vi "rydberg_synth_vi.vi"(8 "error in (no error)":errorcluster, 10 "Novatech Synth Settings":T1[][](array[typedef]) {"Table Mode"."Freq. Step (MHz)" format="%#_9g"; "Table Mode"."FinalFreq" format="%#_9g"; "Table Mode"."Initial Freq.(MHz)" format="%#_9g"; "Channel Settings"."Frequency (MHz)" format="%#_9g"}) -> (0 "error out":errorcluster)   [LabVIEW 2016]
uses:
  Controls/Synth_409b/Synth_controls.ctl
  Controls/Synth_409b/synth_channel.ctl
  Controls/Synth_409b/table_mode.ctl
  <vilib>/Instr/_visa.llb/VISA Configure Serial Port (Instr).vi
panel:
  out "Response":string
  out "Whole Command":string
  # "Red Sat Abs Control - Com 6\nChannel 0: 81.85\nChannel 1: 82.15"
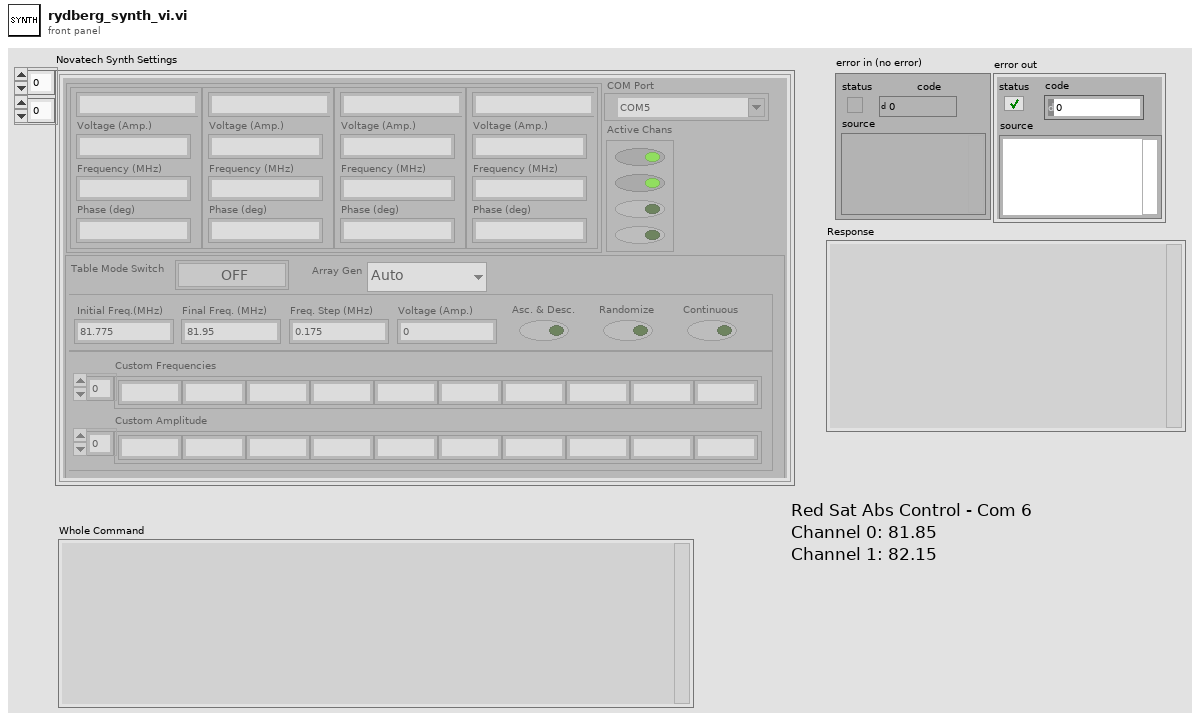
[diagram p1: front panel]
types:
  T1 = typedef "Synth_controls.ctl" = cluster{"Channel Settings":T2[], "Active Chans":bool[], "COM Port":refnum<visa-resource-name>, "Table Mode":T3}
  T2 = typedef "synth_channel.ctl" = cluster{"Voltage (Amp.) ":dbl, "Frequency (MHz)":dbl, "Phase (deg)":dbl, "Nickname":string}
  T3 = typedef "table_mode.ctl" = cluster{"Initial Freq.(MHz)":dbl, "FinalFreq":dbl, "Freq. Step (MHz)":dbl, "Voltage (Amp.)":dbl, "Asc. & Desc.":bool, "Custom Frequencies":dbl[], "Custom Amplitude":dbl[], "Table Mode Switch":bool, "Array Gen":enum16{"Auto", "Custom"}, "Randomize":bool, "Continuous":bool}
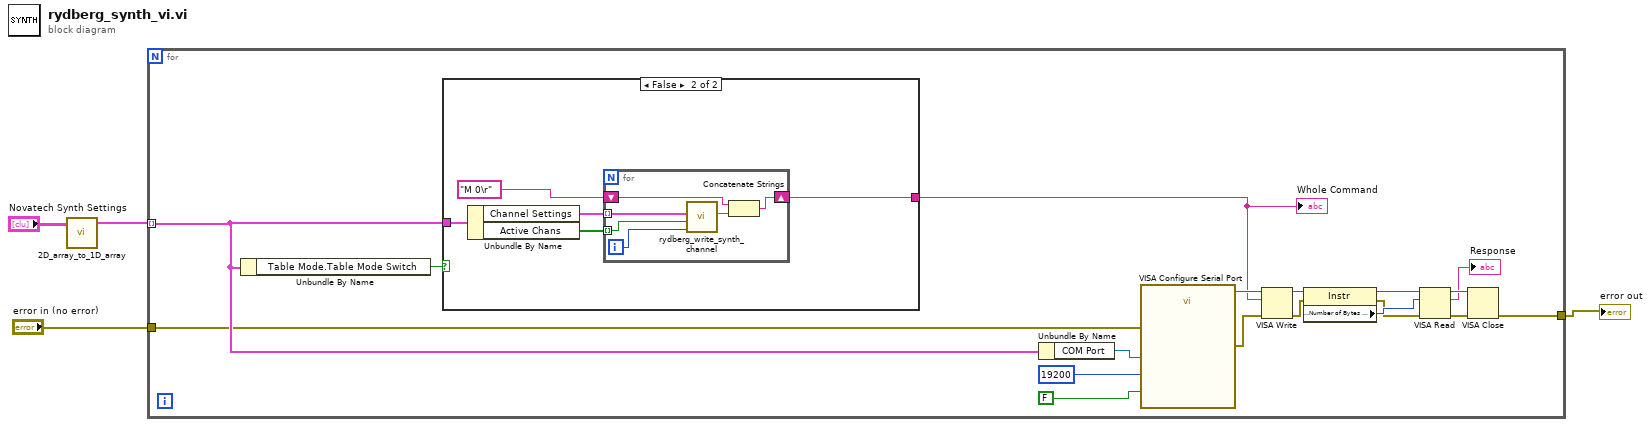
[diagram p0: block diagram]
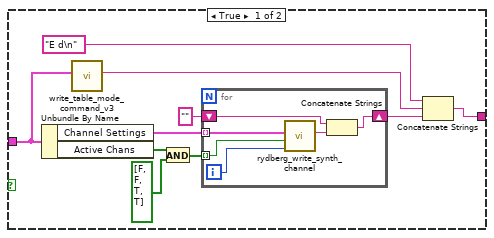
[diagram p2: hidden frame]
diagram:
  n1 = call "2D_array_to_1D_array.vi"("2D Input Arrray"="Novatech Synth Settings") -> ("1D Output array"=w1:T1[])  [unwired: 2 in, 2 out]
  n2 = for {
    tunnel: w1 -> [w7] mode=indexing
    tunnel: "error in (no error)" -> [w6]
    tunnel: [w5] -> w3
    n3 = Unbundle By Name(w7) -> ("Table Mode.Table Mode Switch"=w8:bool)
    n4 = case shown="False" w8 {
      tunnel: w7 -> [w32 w43]
      tunnel: [w29 w39] -> w10
      frame True {
        n5 = Unbundle By Name(w32) -> ("Channel Settings"=w31:T2[], "Active Chans"=w27:bool[])
        n6 = call "write_table_mode_command_v3.vi"("Synth Controls"=w32) -> ("Table Mode Command"=w28:string)  [unwired: 10 in]
        n7 = And(x=w27, y=bool[] [FALSE, FALSE, TRUE, TRUE]) -> (x .and. y?=w25:bool[])
        n8 = for {
          tunnel: w31 -> [w38] mode=indexing
          tunnel: w25 -> [w37] mode=indexing
          shift-right: [w33] -> w30
          shift-left: "" -> [w34]
          i -> [w36]
          n9 = call "rydberg_write_synth_channel.vi"("Channel #"=w36, "Channel Active"=w37, "Channel Parameters"=w38) -> ("Command"=w35:string)  [unwired: 8 in]
          n10 = Concatenate Strings(w34, w35) -> (w33:string)
        }
        n11 = Concatenate Strings("E d\n" ("string"), w28, w30) -> (w29:string)
      }
      frame False {
        n12 = Unbundle By Name(w43) -> ("Channel Settings"=w42:T2[], "Active Chans"=w41:bool[])
        n13 = for {
          tunnel: w42 -> [w49] mode=indexing
          tunnel: w41 -> [w48] mode=indexing
          shift-right: [w44] -> w39
          shift-left: "M 0\r" ("Command") -> [w45]
          i -> [w47]
          n14 = call "rydberg_write_synth_channel.vi"("Channel #"=w47, "Channel Active"=w48, "Channel Parameters"=w49) -> ("Command"=w46:string)  [unwired: 8 in]
          n15 = Concatenate Strings(w45, w46) -> (w44:string)
        }
      }
    }
    "Whole Command" <- w10
    n16 = Unbundle By Name(w7) -> ("COM Port"=w9:refnum<visa-resource-name>)
    n17 = call-poly "VISA Configure Serial Port"("VISA resource name"=w9, "Enable Termination\nChar (T)"=FALSE ("Enable Termination\nChar (T)"), "baud rate (9600)"=u32 19200, "error in (no error)"=w6) -> ("VISA resource name out"=w20:refnum<visa-resource-name>, "error out"=w19:errorcluster)  [unwired: 10 in]
    n18 = VISA Write(VISA resource name=w20, write buffer=w10, error in (no error)=w19) -> (VISA resource name out=w18:refnum<visa-resource-name>, error out=w17:errorcluster)  [unwired: 1 out]
    n19 = property class="Instr"(reference=w18, error in=w17) -> (reference out=w15:refnum<visa-resource-name>, error out=w14:errorcluster, "Serial Settings:Number of Bytes at Serial Port"=w16:u32)
    n20 = VISA Read(VISA resource name=w15, byte count=w16, error in (no error)=w14) -> (VISA resource name out=w13:refnum<visa-resource-name>, read buffer=→"Response":string, error out=w12:errorcluster)  [unwired: 1 out]
    n21 = VISA Close(VISA resource name=w13, error in (no error)=w12) -> (error out=w5:errorcluster)
  }
  "error out" <- w3
